vi "SLM CONTROL v2.vi"() -> ()   [LabVIEW 2014]
panel:
  out "Exit VI 2":bool
  in  "current metric":enum16{"brightness", "sharpness", "both"}(ring)
  in  "holo on 2":bool=TRUE
  in  "holo on 1":bool=TRUE
  in  "discard 1":bool
  in  "correct mode x 1":bool
  in  "mode x 1":i32=5 caption="x"
  in  "align tilt 1":bool
  in  "keep 1":bool
  in  "align tip 1":bool
  in  "discard 2":bool
  in  "correct mode x 2":bool
  in  "mode x 2":i32=5 caption="x"
  in  "align tilt 2":bool
  in  "keep 2":bool
  in  "fitted peak":dbl caption="x"
  in  "loop index":i32 caption="x"
  out "Metric Plots":cluster{dbl[], dbl[]}[](graph)
  in  "S Max":dbl=0.2 caption="x"
  in  "M":dbl[](array[numeric])=[0.0, 0.0]
  in  "BG Offset":dbl=0.2 caption="x"
  in  "Rmask":dbl=0.2 caption="x"
  in  "I":dbl[](array[numeric])=[0.0, 0.0, 0.0, 0.0, 0.0]
  in  "S":dbl[](array[numeric])=[0.0, 0.0, 0.0, 0.0, 0.0]
  in  "resolution":dbl=0.2 caption="x"
  out "current mode number":i32=5 caption="x"
  out "current holo number":i32=2 caption="x"
  in  "alignment offset":dbl[](array[numeric])=[0.0, 0.0]
  in  "step size align":dbl=0.2 caption="step size"
  in  "number of steps align":i32=3 caption="# steps"
  in  "align tip 2":bool
  in  "load BMP":bool
  in  "save hologram":bool
  in  "top hat radius":dbl=0.66
  out "mode matrix name":string="Unit Matrix.csv"
  in  "set mode matrix name":bool
  in  "holo size":i32=300
  in  "wrap value":i32=20
  in  "SLM number":i32=197
  in  "apply flatness":bool
  out "hologram":u8[][](graph)
  in  "vortex dir 2":bool
  in  "vortex dir 1":bool
  in  "top hat 2":bool
  in  "vortex 2":bool
  in  "top hat 1":bool
  in  "vortex 1":bool
  in  "holo y pos 2":dbl caption="y"
  in  "holo x pos 2":dbl=200.0 caption="x"
  in  "holo y pos 1":dbl caption="y"
  in  "holo x pos 1":dbl=-200.0 caption="x"
  in  "background gradient y":dbl=-40.0 caption="y"
  in  "background gradient x":dbl=-40.0 caption="x"
  in  "merlin coefficients 2":dbl[][](array[numeric])=[[0.0, 0.0], [0.0, 0.0], [0.0, 0.0]]
  in  "routine coefficients 2":dbl[][](array[numeric])=[[0.0, 0.0], [0.0, 0.0], [0.0, 0.0]]
  in  "manual coefficients 2":dbl[][](array[numeric])=[[2.0, 0.0], [3.0, 0.0], [4.0, 1.0]]
  in  "grating coefficients 2":dbl[][](array[numeric])=[[2.0, 0.0], [3.0, 0.0]]
  in  "merlin coefficients 1":dbl[][](array[numeric])=[[0.0, 0.0], [0.0, 0.0], [0.0, 0.0]]
  in  "routine coefficients 1":dbl[][](array[numeric])=[[0.0, 0.0], [0.0, 0.0], [0.0, 0.0]]
  in  "manual coefficients 1":dbl[][](array[numeric])=[[2.0, 0.0], [3.0, 0.0], [4.0, 1.0]]
  in  "grating coefficients 1":dbl[][](array[numeric])=[[2.0, 0.0], [3.0, 0.0]]
  in  "modes in memory":i32=20 caption="# modes"
  in  "wavelength (nm)":i32=197
  in  "max wavelength (nm)":i32=800
  in  "min wavelength (nm)":i32=700
  out "root path":path
  out "Sub VI Ready?":bool
  in  "Exit VI":bool
  # "Holo 1"
  # "Holo 2"
  # "Background"
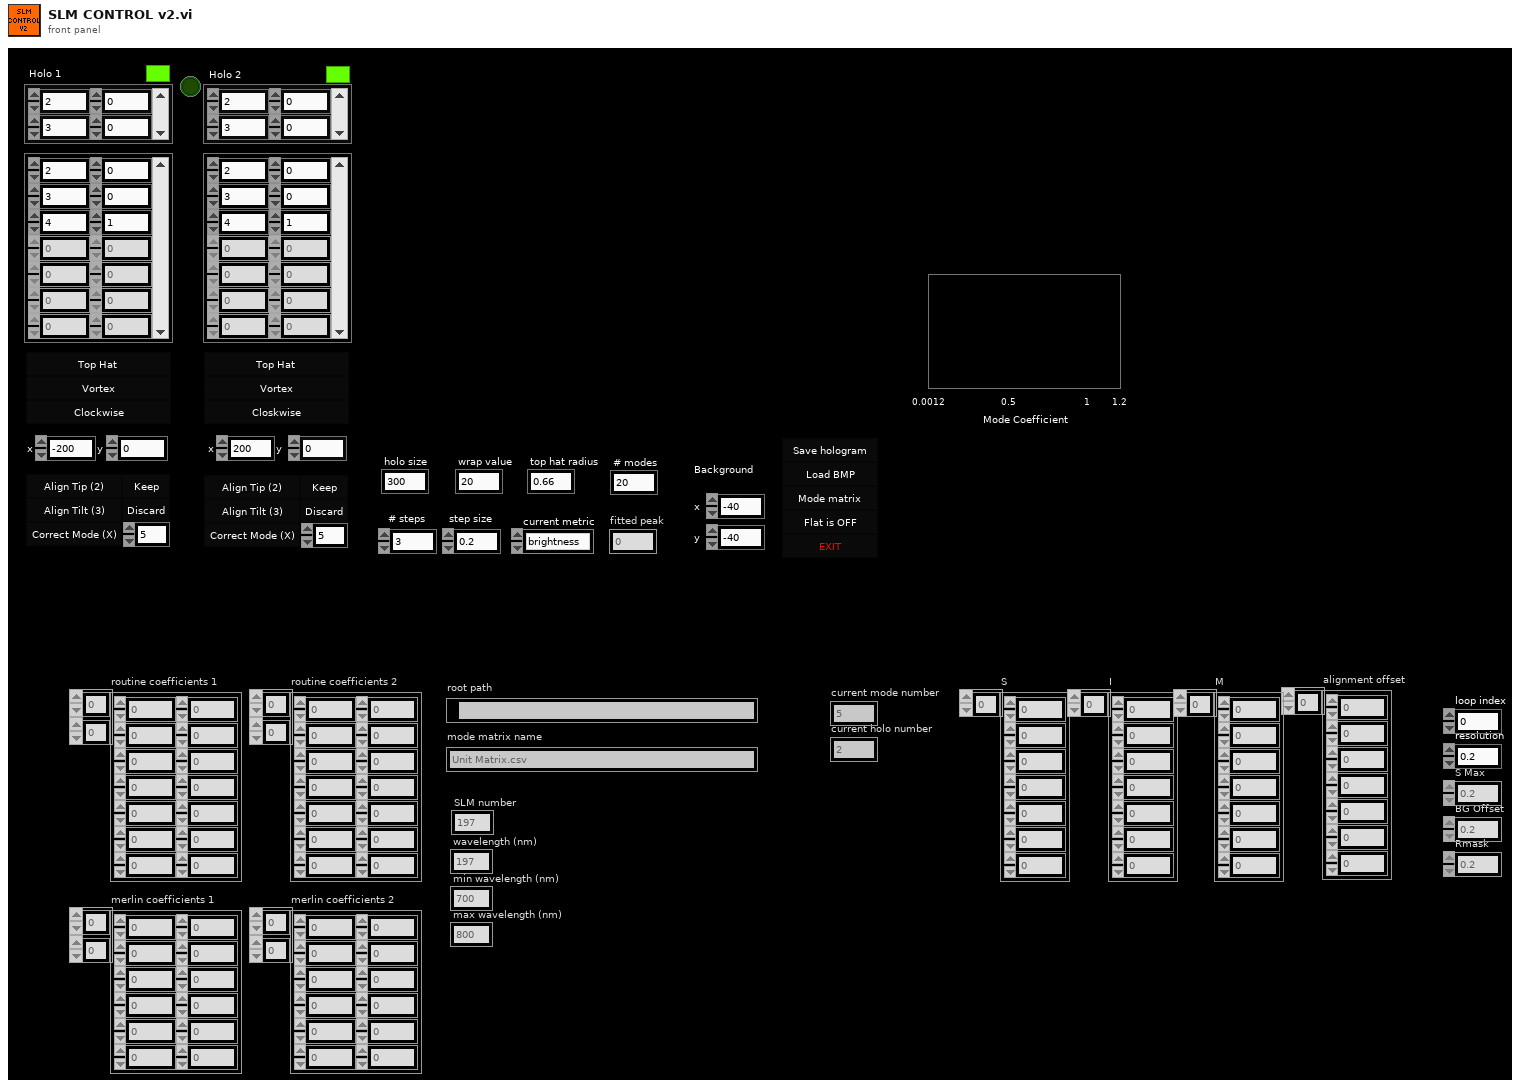
[diagram p1: front panel]
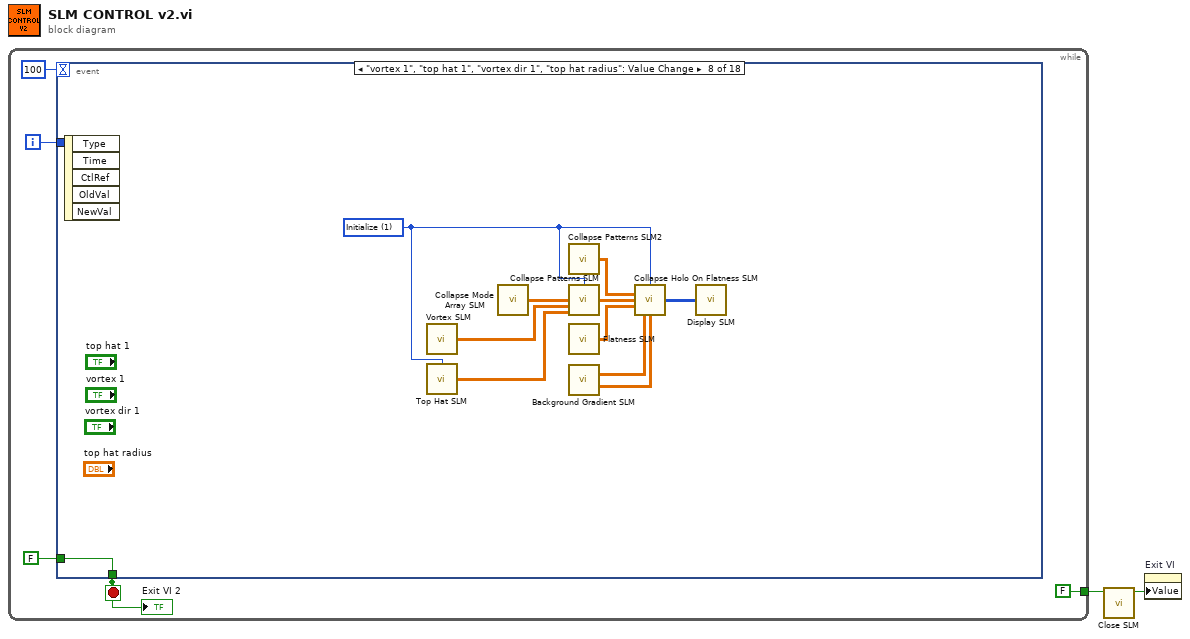
[diagram p0: block diagram]
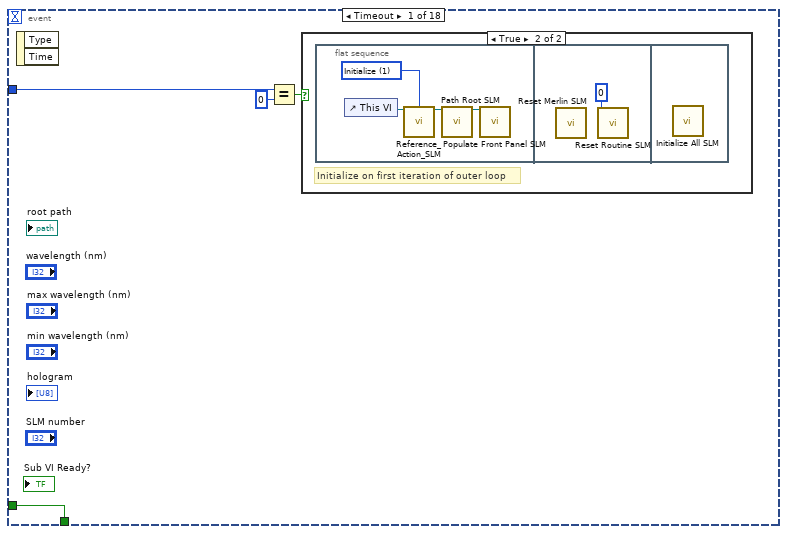
[diagram p2: hidden frame]
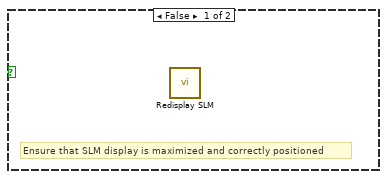
[diagram p3: hidden frame]
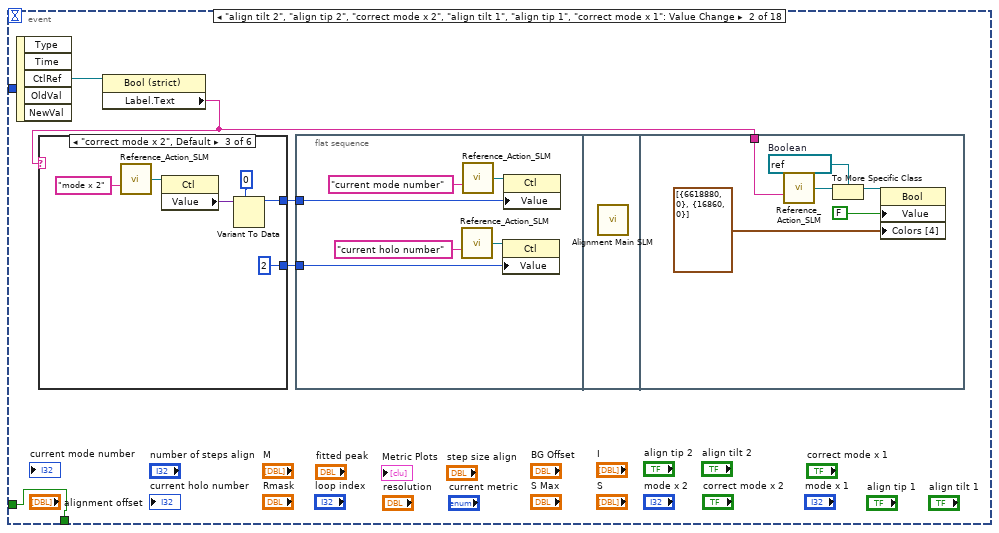
[diagram p4: hidden frame]
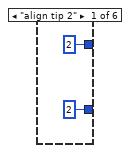
[diagram p5: hidden frame]
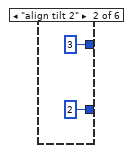
[diagram p6: hidden frame]
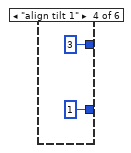
[diagram p7: hidden frame]
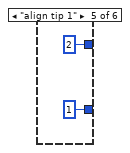
[diagram p8: hidden frame]
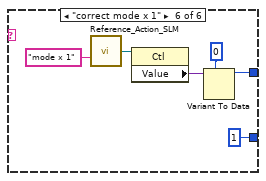
[diagram p9: hidden frame]
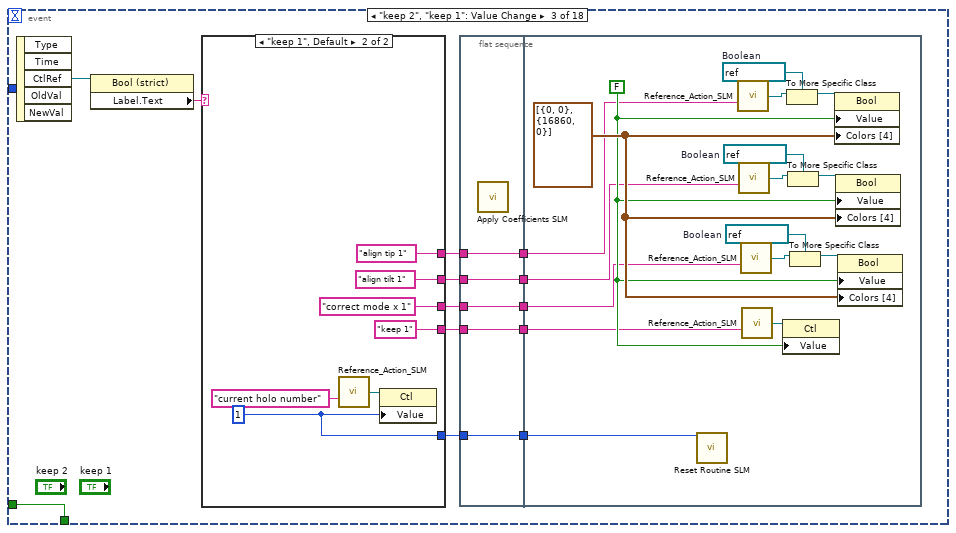
[diagram p10: hidden frame]
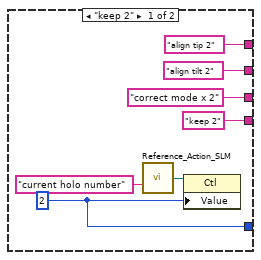
[diagram p11: hidden frame]
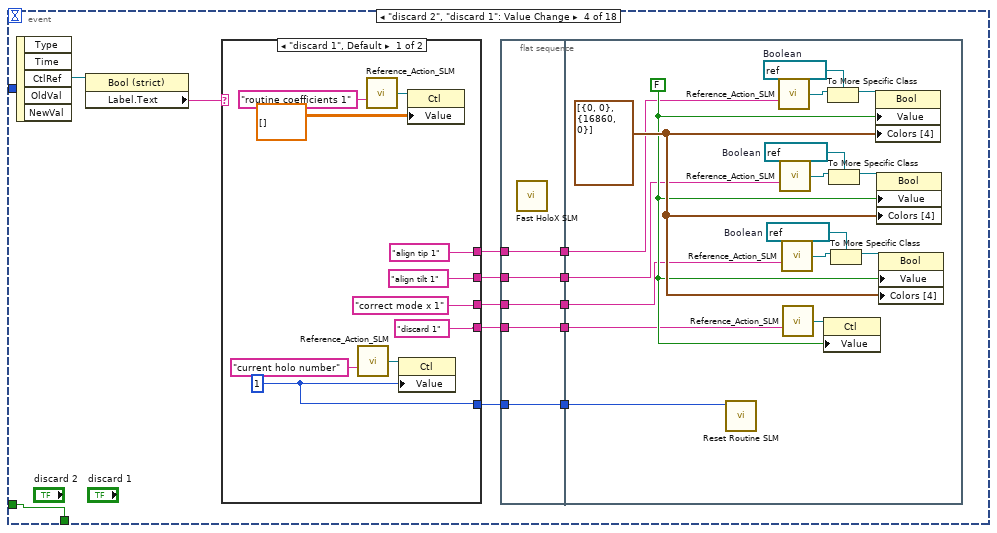
[diagram p12: hidden frame]
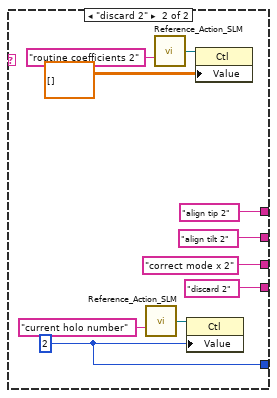
[diagram p13: hidden frame]
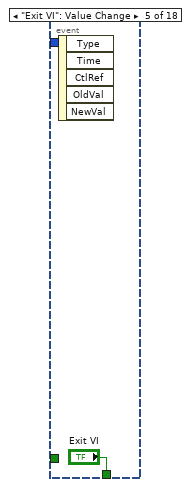
[diagram p14: hidden frame]
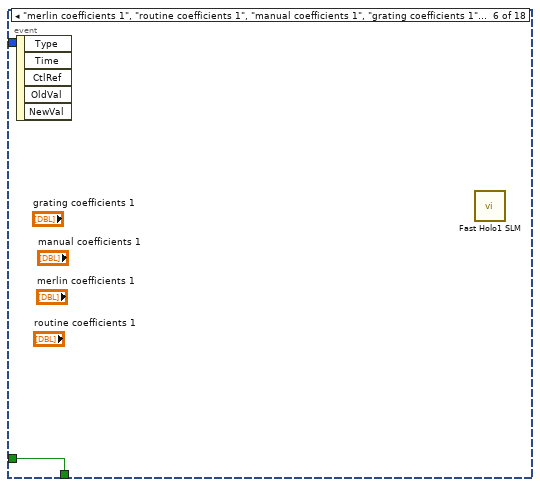
[diagram p15: hidden frame]
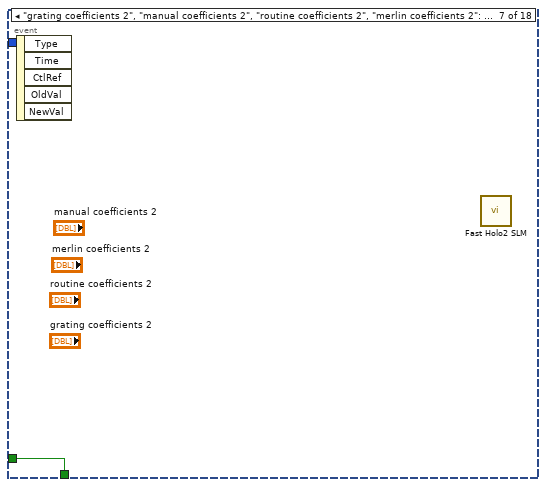
[diagram p16: hidden frame]
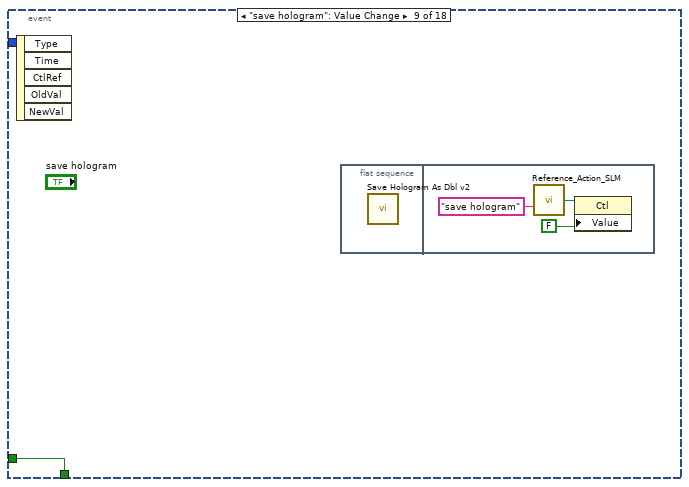
[diagram p17: hidden frame]
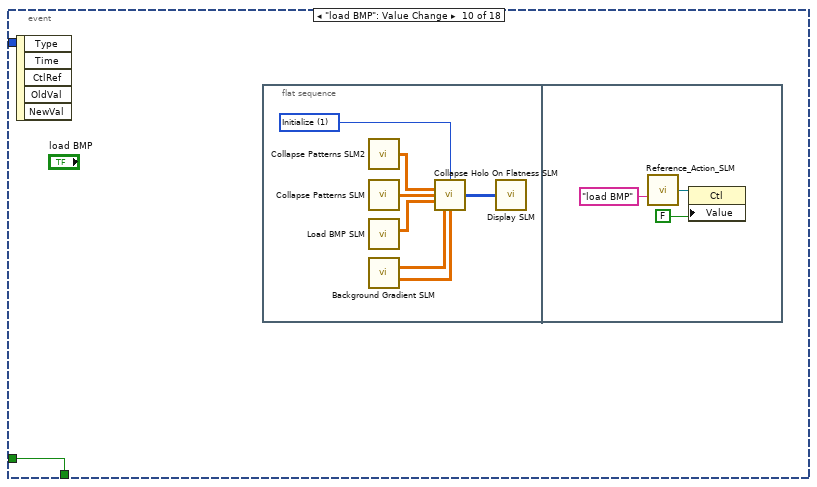
[diagram p18: hidden frame]
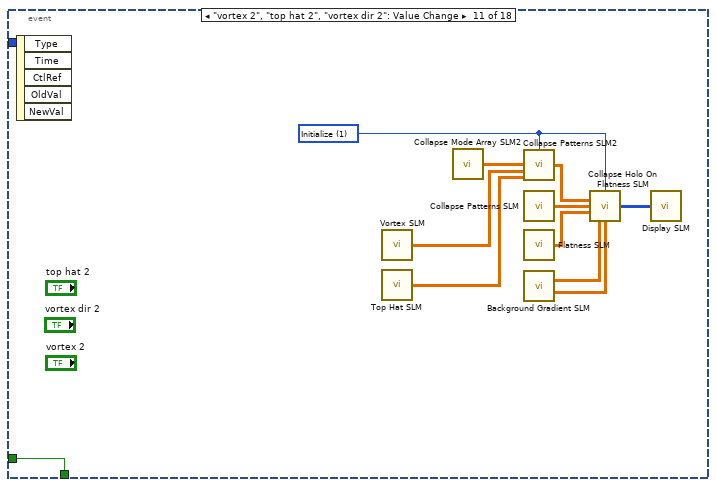
[diagram p19: hidden frame]
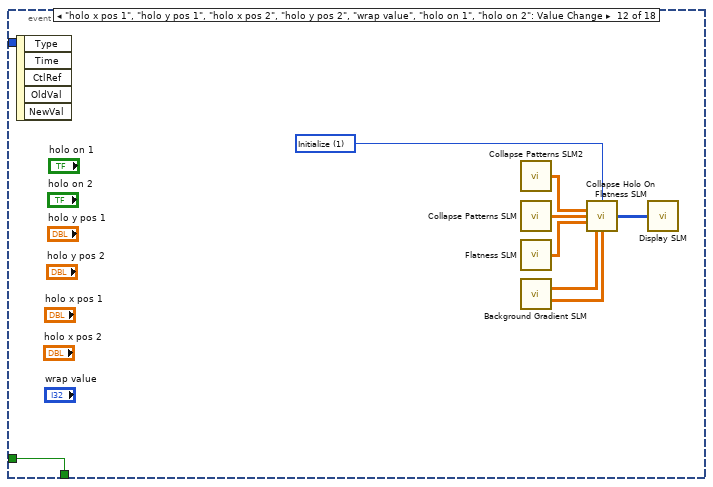
[diagram p20: hidden frame]
diagram:
  n1 = while {
    tunnel: [FALSE] -> w2
    i -> [w4]
    stop <- w7 stop-if-true
    n2 = event shown="[7] \"vortex 1\", \"top hat 1\", \"vortex dir 1\", \"top hat radius\": Value Change" {
      selector: _ -> [_ _ _ _ _ _ _ _ _ _ _ _ _ _ _ _ _ _]
      dyn-events: _ -> [_ _ _ _ _ _ _ _ _ _ _ _ _ _ _ _ _ _]
      timeout: 100 -> [_ _ _ _ _ _ _ _ _ _ _ _ _ _ _ _ _ _]
      tunnel: [w11 w17 w54 w103 "Exit VI" w159 w160 w161 w172 w176 w187 w198 w206 w214 w222 w235 w239 w244] -> w7
      tunnel: FALSE -> [w11 w17 w54 w103 _ w159 w160 w161 w172 w176 w187 w198 w206 w214 w222 w235 w239 w244]
      tunnel: w4 -> [w8 _ _ _ _ _ _ _ _ _ _ _ _ _ _ _ _ _]
      event Timeout {
        n3 = event-data() -> ()  [unwired: 3 out]
        n4 = Equal?(x=w8, y=0) -> (x = y?=w9:bool)
        n5 = case shown="True" w9 {
          frame False {
            # "Ensure that SLM display is maximized and correctly positioned"
            n6 = call "Redisplay SLM.vi"() -> ()  [unwired: 12 in]
          }
          frame True {
            # "Initialize on first iteration of outer loop"
            n7 = flat-sequence {
              frame #0 {
                w14 = u16 1 items=["Read", "Initialize"] ("Action")
                n8 = control-ref of="This VI"() -> (w13:refnum<vi>)
                n9 = call "Reference_Action_SLM.vi"("VI Ref IN"=w13, "Action"=w14) -> ("VI Reference"=w15:refnum<vi>)  [unwired: 11 in, 2 out]
                n10 = call "Path Root SLM.vi"("VI Ref IN"=w15) -> ("VI Ref OUT"=w12:refnum<vi>)  [unwired: 14 in]
                n11 = call "Populate Front Panel SLM.vi"("This VI"=w12) -> ()  [unwired: 11 in]
              }
              frame #1 {
                n12 = call "Reset Merlin SLM.vi"() -> ()  [unwired: 12 in]
                n13 = call "Reset Routine SLM.vi"("Numeric"=0) -> ()  [unwired: 11 in]
              }
              frame #2 {
                n14 = call "Initialize All SLM.vi"() -> ()  [unwired: 16 in]
              }
            }
          }
        }
      }
      event "align tilt 2", "align tip 2", "correct mode x 2", "align tilt 1", "align tip 1", "correct mode x 1": Value Change {
        n15 = event-data() -> ("CtlRef"=w21:refnum<vi>)  [unwired: 5 out]
        n16 = property class="Bool (strict)"(reference=w21) -> ("Label.Text"=w18:string)  [unwired: 1 in, 2 out]
        n17 = case shown="\"correct mode x 2\", Default" w18 {
          tunnel: [2 2 2 1 1 1] -> w20
          tunnel: [2 3 w27 3 2 w37] -> w19
          frame "align tip 2" {
          }
          frame "align tilt 2" {
          }
          frame "correct mode x 2", Default {
            n18 = call "Reference_Action_SLM.vi"("Control Name"="mode x 2") -> ("Ref OUT"=w29:refnum<vi>)  [unwired: 12 in, 2 out]
            n19 = property class="Ctl"(reference=w29) -> ("Value"=w30:variant)  [unwired: 1 in, 2 out]
            n20 = Variant To Data(type=0, Variant=w30) -> (data=w27:i32)  [unwired: 1 in, 1 out]
          }
          frame "align tilt 1" {
          }
          frame "align tip 1" {
          }
          frame "correct mode x 1" {
            n21 = call "Reference_Action_SLM.vi"("Control Name"="mode x 1") -> ("Ref OUT"=w39:refnum<vi>)  [unwired: 12 in, 2 out]
            n22 = property class="Ctl"(reference=w39) -> ("Value"=w40:variant)  [unwired: 1 in, 2 out]
            n23 = Variant To Data(type=0, Variant=w40) -> (data=w37:i32)  [unwired: 1 in, 1 out]
          }
        }
        n24 = flat-sequence {
          tunnel: w20 -> [w43]
          tunnel: w19 -> [w42]
          tunnel: w18 -> [w48]
          frame #0 {
            n25 = call "Reference_Action_SLM.vi"("Control Name"="current holo number") -> ("Ref OUT"=w44:refnum<vi>)  [unwired: 12 in, 2 out]
            n26 = call "Reference_Action_SLM.vi"("Control Name"="current mode number") -> ("Ref OUT"=w46:refnum<vi>)  [unwired: 12 in, 2 out]
            n27 = property class="Ctl"(reference=w44, "Value"=w43) -> ()  [unwired: 1 in, 2 out]
            n28 = property class="Ctl"(reference=w46, "Value"=w42) -> ()  [unwired: 1 in, 2 out]
          }
          frame #1 {
            n29 = call "Alignment Main SLM.vi"() -> ()  [unwired: 12 in]
          }
          frame #2 {
            w51 = refnum<vi> refnum  # Boolean
            n30 = call "Reference_Action_SLM.vi"("Control Name"=w48) -> ("Ref OUT"=w53:refnum<vi>)  [unwired: 12 in, 2 out]
            n31 = To More Specific Class(target class=w51, reference=w53) -> (specific class reference=w52:refnum<vi>)  [unwired: 1 in, 1 out]
            n32 = property class="Bool"(reference=w52, "Value"=FALSE, "Colors [4]"=cluster{u32, u32}[] [{6618880, 0}, {16860, 0}]) -> ()  [unwired: 1 in, 2 out]
          }
        }
      }
      event "keep 2", "keep 1": Value Change {
        n33 = event-data() -> ("CtlRef"=w66:refnum<vi>)  [unwired: 5 out]
        n34 = property class="Bool (strict)"(reference=w66) -> ("Label.Text"=w65:string)  [unwired: 1 in, 2 out]
        n35 = case shown="\"keep 1\", Default" w65 {
          tunnel: ["keep 2" ("Control Name") "keep 1" ("Control Name")] -> w63
          tunnel: ["correct mode x 2" ("Control Name") "correct mode x 1" ("Control Name")] -> w61
          tunnel: ["align tilt 2" ("Control Name") "align tilt 1" ("Control Name")] -> w59
          tunnel: ["align tip 2" ("Control Name") "align tip 1" ("Control Name")] -> w57
          tunnel: [w67 w74] -> w55
          frame "keep 2" {
            w67 = 2
            n36 = call "Reference_Action_SLM.vi"("Control Name"="current holo number") -> ("Ref OUT"=w69:refnum<vi>)  [unwired: 12 in, 2 out]
            n37 = property class="Ctl"(reference=w69, "Value"=w67) -> ()  [unwired: 1 in, 2 out]
          }
          frame "keep 1", Default {
            w74 = 1
            n38 = call "Reference_Action_SLM.vi"("Control Name"="current holo number") -> ("Ref OUT"=w76:refnum<vi>)  [unwired: 12 in, 2 out]
            n39 = property class="Ctl"(reference=w76, "Value"=w74) -> ()  [unwired: 1 in, 2 out]
          }
        }
        n40 = flat-sequence {
          tunnel: [w85] -> w64
          tunnel: w63 -> [w85]
          tunnel: [w84] -> w62
          tunnel: w61 -> [w84]
          tunnel: [w83] -> w60
          tunnel: w59 -> [w83]
          tunnel: [w82] -> w58
          tunnel: w57 -> [w82]
          tunnel: [w81] -> w56
          tunnel: w55 -> [w81]
          tunnel: w64 -> [w90]
          tunnel: w62 -> [w89]
          tunnel: w60 -> [w88]
          tunnel: w58 -> [w87]
          tunnel: w56 -> [w86]
          frame #0 {
            n41 = call "Apply Coefficients SLM.vi"() -> ()  [unwired: 12 in]
          }
          frame #1 {
            w93 = refnum<vi> refnum  # Boolean
            w92 = cluster{u32, u32}[] [{0, 0}, {16860, 0}] ("Colors [4]")
            w96 = refnum<vi> refnum  # Boolean
            w91 = FALSE
            w99 = refnum<vi> refnum  # Boolean
            n42 = call "Reset Routine SLM.vi"("Numeric"=w86) -> ()  [unwired: 11 in]
            n43 = call "Reference_Action_SLM.vi"("Control Name"=w87) -> ("Ref OUT"=w101:refnum<vi>)  [unwired: 12 in, 2 out]
            n44 = call "Reference_Action_SLM.vi"("Control Name"=w88) -> ("Ref OUT"=w98:refnum<vi>)  [unwired: 12 in, 2 out]
            n45 = call "Reference_Action_SLM.vi"("Control Name"=w89) -> ("Ref OUT"=w95:refnum<vi>)  [unwired: 12 in, 2 out]
            n46 = call "Reference_Action_SLM.vi"("Control Name"=w90) -> ("Ref OUT"=w102:refnum<vi>)  [unwired: 12 in, 2 out]
            n47 = property class="Ctl"(reference=w102, "Value"=w91) -> ()  [unwired: 1 in, 2 out]
            n48 = To More Specific Class(target class=w99, reference=w101) -> (specific class reference=w100:refnum<vi>)  [unwired: 1 in, 1 out]
            n49 = To More Specific Class(target class=w96, reference=w98) -> (specific class reference=w97:refnum<vi>)  [unwired: 1 in, 1 out]
            n50 = To More Specific Class(target class=w93, reference=w95) -> (specific class reference=w94:refnum<vi>)  [unwired: 1 in, 1 out]
            n51 = property class="Bool"(reference=w100, "Value"=w91, "Colors [4]"=w92) -> ()  [unwired: 1 in, 2 out]
            n52 = property class="Bool"(reference=w97, "Value"=w91, "Colors [4]"=w92) -> ()  [unwired: 1 in, 2 out]
            n53 = property class="Bool"(reference=w94, "Value"=w91, "Colors [4]"=w92) -> ()  [unwired: 1 in, 2 out]
          }
        }
      }
      event "discard 2", "discard 1": Value Change {
        n54 = event-data() -> ("CtlRef"=w115:refnum<vi>)  [unwired: 5 out]
        n55 = property class="Bool (strict)"(reference=w115) -> ("Label.Text"=w114:string)  [unwired: 1 in, 2 out]
        n56 = case shown="\"discard 1\", Default" w114 {
          tunnel: ["discard 1" ("Control Name") "discard 2" ("Control Name")] -> w106
          tunnel: ["correct mode x 1" ("Control Name") "correct mode x 2" ("Control Name")] -> w107
          tunnel: ["align tilt 1" ("Control Name") "align tilt 2" ("Control Name")] -> w108
          tunnel: ["align tip 1" ("Control Name") "align tip 2" ("Control Name")] -> w109
          tunnel: [w138 w148] -> w104
          frame "discard 1", Default {
            w138 = 1
            n57 = call "Reference_Action_SLM.vi"("Control Name"="current holo number") -> ("Ref OUT"=w144:refnum<vi>)  [unwired: 12 in, 2 out]
            n58 = call "Reference_Action_SLM.vi"("Control Name"="routine coefficients 1") -> ("Ref OUT"=w145:refnum<vi>)  [unwired: 12 in, 2 out]
            n59 = property class="Ctl"(reference=w144, "Value"=w138) -> ()  [unwired: 1 in, 2 out]
            n60 = property class="Ctl"(reference=w145, "Value"=dbl[][] [] ("routine coefficients 2")) -> ()  [unwired: 1 in, 2 out]
          }
          frame "discard 2" {
            w148 = 2
            n61 = call "Reference_Action_SLM.vi"("Control Name"="current holo number") -> ("Ref OUT"=w150:refnum<vi>)  [unwired: 12 in, 2 out]
            n62 = call "Reference_Action_SLM.vi"("Control Name"="routine coefficients 2") -> ("Ref OUT"=w151:refnum<vi>)  [unwired: 12 in, 2 out]
            n63 = property class="Ctl"(reference=w150, "Value"=w148) -> ()  [unwired: 1 in, 2 out]
            n64 = property class="Ctl"(reference=w151, "Value"=dbl[][] [] ("routine coefficients 2")) -> ()  [unwired: 1 in, 2 out]
          }
        }
        n65 = flat-sequence {
          tunnel: [w120] -> w113
          tunnel: w106 -> [w120]
          tunnel: [w119] -> w112
          tunnel: w107 -> [w119]
          tunnel: [w118] -> w111
          tunnel: w108 -> [w118]
          tunnel: [w117] -> w110
          tunnel: w109 -> [w117]
          tunnel: [w116] -> w105
          tunnel: w104 -> [w116]
          tunnel: w113 -> [w125]
          tunnel: w112 -> [w124]
          tunnel: w111 -> [w123]
          tunnel: w110 -> [w122]
          tunnel: w105 -> [w121]
          frame #0 {
            n66 = call "Fast HoloX SLM.vi"() -> ()  [unwired: 12 in]
          }
          frame #1 {
            w128 = refnum<vi> refnum  # Boolean
            w127 = cluster{u32, u32}[] [{0, 0}, {16860, 0}] ("Colors [4]")
            w131 = refnum<vi> refnum  # Boolean
            w126 = FALSE
            w134 = refnum<vi> refnum  # Boolean
            n67 = call "Reset Routine SLM.vi"("Numeric"=w121) -> ()  [unwired: 11 in]
            n68 = call "Reference_Action_SLM.vi"("Control Name"=w122) -> ("Ref OUT"=w136:refnum<vi>)  [unwired: 12 in, 2 out]
            n69 = call "Reference_Action_SLM.vi"("Control Name"=w123) -> ("Ref OUT"=w133:refnum<vi>)  [unwired: 12 in, 2 out]
            n70 = call "Reference_Action_SLM.vi"("Control Name"=w124) -> ("Ref OUT"=w130:refnum<vi>)  [unwired: 12 in, 2 out]
            n71 = call "Reference_Action_SLM.vi"("Control Name"=w125) -> ("Ref OUT"=w137:refnum<vi>)  [unwired: 12 in, 2 out]
            n72 = property class="Ctl"(reference=w137, "Value"=w126) -> ()  [unwired: 1 in, 2 out]
            n73 = To More Specific Class(target class=w134, reference=w136) -> (specific class reference=w135:refnum<vi>)  [unwired: 1 in, 1 out]
            n74 = To More Specific Class(target class=w131, reference=w133) -> (specific class reference=w132:refnum<vi>)  [unwired: 1 in, 1 out]
            n75 = To More Specific Class(target class=w128, reference=w130) -> (specific class reference=w129:refnum<vi>)  [unwired: 1 in, 1 out]
            n76 = property class="Bool"(reference=w135, "Value"=w126, "Colors [4]"=w127) -> ()  [unwired: 1 in, 2 out]
            n77 = property class="Bool"(reference=w132, "Value"=w126, "Colors [4]"=w127) -> ()  [unwired: 1 in, 2 out]
            n78 = property class="Bool"(reference=w129, "Value"=w126, "Colors [4]"=w127) -> ()  [unwired: 1 in, 2 out]
          }
        }
      }
      event "Exit VI": Value Change {
        n79 = event-data() -> ()  [unwired: 6 out]
      }
      event "merlin coefficients 1", "routine coefficients 1", "manual coefficients 1", "grating coefficients 1": Value Change {
        n80 = event-data() -> ()  [unwired: 6 out]
        n81 = call "Fast Holo1 SLM.vi"() -> ()  [unwired: 12 in]
      }
      event "grating coefficients 2", "manual coefficients 2", "routine coefficients 2", "merlin coefficients 2": Value Change {
        n82 = event-data() -> ()  [unwired: 6 out]
        n83 = call "Fast Holo2 SLM.vi"() -> ()  [unwired: 12 in]
      }
      event "vortex 1", "top hat 1", "vortex dir 1", "top hat radius": Value Change {
        w162 = u16 1 items=["Read", "Initialize"] ("Action")
        n84 = event-data() -> ()  [unwired: 6 out]
        n85 = call "Vortex SLM.vi"() -> ("Vortex"=w169:dbl[][])  [unwired: 15 in]
        n86 = call "Top Hat SLM.vi"("Action"=w162) -> ("Top hat"=w168:dbl[][])  [unwired: 14 in]
        n87 = call "Collapse Mode Array SLM.vi"() -> ("collapsed mode array"=w171:dbl[][])  [unwired: 15 in]
        n88 = call "Collapse Patterns SLM2.vi"() -> ("collapsed patterns"=w165:dbl[][])  [unwired: 15 in]
        n89 = call "Collapse Patterns SLM.vi"("Action"=w162, "collapsed mode array"=w171, "Vortex"=w169, "Top hat"=w168) -> ("collapsed patterns"=w170:dbl[][])  [unwired: 11 in]
        n90 = call "Flatness SLM.vi"() -> ("flatness"=w167:dbl[][])  [unwired: 15 in]
        n91 = call "Background Gradient SLM.vi"() -> ("gradient"=w164:dbl[][], "holo mask"=w163:dbl[][])  [unwired: 14 in]
        n92 = call "Collapse Holo On Flatness SLM.vi"("Action"=w162, "collapsed patterns 2"=w165, "collapsed patterns"=w170, "flatness"=w167, "gradient"=w164, "holo mask"=w163) -> ("displayed matrix"=w166:u8[][])  [unwired: 9 in]
        n93 = call "Display SLM.vi"("displayed matrix"=w166) -> ()  [unwired: 14 in, 1 out]
      }
      event "save hologram": Value Change {
        n94 = event-data() -> ()  [unwired: 6 out]
        n95 = flat-sequence {
          frame #0 {
            n96 = call "Save Hologram As Dbl v2.vi"() -> ()  [unwired: 12 in]
          }
          frame #1 {
            n97 = call "Reference_Action_SLM.vi"("Control Name"="save hologram") -> ("Ref OUT"=w174:refnum<vi>)  [unwired: 12 in, 2 out]
            n98 = property class="Ctl"(reference=w174, "Value"=FALSE ("Load Matrix")) -> ()  [unwired: 1 in, 2 out]
          }
        }
      }
      event "load BMP": Value Change {
        n99 = event-data() -> ()  [unwired: 6 out]
        n100 = flat-sequence {
          frame #0 {
            w178 = u16 1 items=["Read", "Initialize"] ("Action")
            n101 = call "Collapse Patterns SLM2.vi"() -> ("collapsed patterns"=w181:dbl[][])  [unwired: 15 in]
            n102 = call "Collapse Patterns SLM.vi"() -> ("collapsed patterns"=w183:dbl[][])  [unwired: 15 in]
            n103 = call "Load BMP SLM.vi"() -> ("double precision float"=w177:dbl[][])  [unwired: 11 in]
            n104 = call "Background Gradient SLM.vi"() -> ("gradient"=w180:dbl[][], "holo mask"=w179:dbl[][])  [unwired: 14 in]
            n105 = call "Collapse Holo On Flatness SLM.vi"("Action"=w178, "collapsed patterns 2"=w181, "collapsed patterns"=w183, "flatness"=w177, "gradient"=w180, "holo mask"=w179) -> ("displayed matrix"=w182:u8[][])  [unwired: 9 in]
            n106 = call "Display SLM.vi"("displayed matrix"=w182) -> ()  [unwired: 14 in, 1 out]
          }
          frame #1 {
            n107 = call "Reference_Action_SLM.vi"("Control Name"="load BMP") -> ("Ref OUT"=w185:refnum<vi>)  [unwired: 12 in, 2 out]
            n108 = property class="Ctl"(reference=w185, "Value"=FALSE ("Load Matrix")) -> ()  [unwired: 1 in, 2 out]
          }
        }
      }
      event "vortex 2", "top hat 2", "vortex dir 2": Value Change {
        w193 = u16 1 items=["Read", "Initialize"] ("Action")
        n109 = event-data() -> ()  [unwired: 6 out]
        n110 = call "Vortex SLM.vi"() -> ("Vortex"=w191:dbl[][])  [unwired: 15 in]
        n111 = call "Top Hat SLM.vi"() -> ("Top hat"=w190:dbl[][])  [unwired: 15 in]
        n112 = call "Collapse Mode Array SLM2.vi"() -> ("collapsed mode array"=w192:dbl[][])  [unwired: 15 in]
        n113 = call "Collapse Patterns SLM2.vi"("Action"=w193, "collapsed mode array"=w192, "Vortex"=w191, "Top hat"=w190) -> ("collapsed patterns"=w194:dbl[][])  [unwired: 11 in]
        n114 = call "Collapse Patterns SLM.vi"() -> ("collapsed patterns"=w197:dbl[][])  [unwired: 15 in]
        n115 = call "Flatness SLM.vi"() -> ("flatness"=w196:dbl[][])  [unwired: 15 in]
        n116 = call "Background Gradient SLM.vi"() -> ("gradient"=w189:dbl[][], "holo mask"=w188:dbl[][])  [unwired: 14 in]
        n117 = call "Collapse Holo On Flatness SLM.vi"("Action"=w193, "collapsed patterns 2"=w194, "collapsed patterns"=w197, "flatness"=w196, "gradient"=w189, "holo mask"=w188) -> ("displayed matrix"=w195:u8[][])  [unwired: 9 in]
        n118 = call "Display SLM.vi"("displayed matrix"=w195) -> ()  [unwired: 14 in, 1 out]
      }
      event "holo x pos 1", "holo y pos 1", "holo x pos 2", "holo y pos 2", "wrap value", "holo on 1", "holo on 2": Value Change {
        w205 = u16 1 items=["Read", "Initialize"] ("Action")
        n119 = event-data() -> ()  [unwired: 6 out]
        n120 = call "Collapse Patterns SLM2.vi"() -> ("collapsed patterns"=w201:dbl[][])  [unwired: 15 in]
        n121 = call "Collapse Patterns SLM.vi"() -> ("collapsed patterns"=w202:dbl[][])  [unwired: 15 in]
        n122 = call "Flatness SLM.vi"() -> ("flatness"=w203:dbl[][])  [unwired: 15 in]
        n123 = call "Background Gradient SLM.vi"() -> ("gradient"=w200:dbl[][], "holo mask"=w199:dbl[][])  [unwired: 14 in]
        n124 = call "Collapse Holo On Flatness SLM.vi"("Action"=w205, "collapsed patterns 2"=w201, "collapsed patterns"=w202, "flatness"=w203, "gradient"=w200, "holo mask"=w199) -> ("displayed matrix"=w204:u8[][])  [unwired: 9 in]
        n125 = call "Display SLM.vi"("displayed matrix"=w204) -> ()  [unwired: 14 in, 1 out]
      }
      event "background gradient x", "background gradient y": Value Change {
        w208 = u16 1 items=["Read", "Initialize"] ("Action")
        n126 = event-data() -> ()  [unwired: 6 out]
        n127 = call "Collapse Patterns SLM2.vi"() -> ("collapsed patterns"=w210:dbl[][])  [unwired: 15 in]
        n128 = call "Collapse Patterns SLM.vi"() -> ("collapsed patterns"=w211:dbl[][])  [unwired: 15 in]
        n129 = call "Flatness SLM.vi"() -> ("flatness"=w212:dbl[][])  [unwired: 15 in]
        n130 = call "Background Gradient SLM.vi"("Action"=w208) -> ("gradient"=w209:dbl[][], "holo mask"=w207:dbl[][])  [unwired: 13 in]
        n131 = call "Collapse Holo On Flatness SLM.vi"("Action"=w208, "collapsed patterns 2"=w210, "collapsed patterns"=w211, "flatness"=w212, "gradient"=w209, "holo mask"=w207) -> ("displayed matrix"=w213:u8[][])  [unwired: 9 in]
        n132 = call "Display SLM.vi"("displayed matrix"=w213) -> ()  [unwired: 14 in, 1 out]
      }
      event "apply flatness": Value Change {
        w215 = u16 1 items=["Read", "Initialize"] ("Action")
        n133 = event-data() -> ()  [unwired: 6 out]
        n134 = call "Collapse Patterns SLM2.vi"() -> ("collapsed patterns"=w218:dbl[][])  [unwired: 15 in]
        n135 = call "Collapse Patterns SLM.vi"() -> ("collapsed patterns"=w219:dbl[][])  [unwired: 15 in]
        n136 = call "Flatness SLM.vi"("Action"=w215) -> ("flatness"=w220:dbl[][])  [unwired: 14 in]
        n137 = call "Background Gradient SLM.vi"() -> ("gradient"=w217:dbl[][], "holo mask"=w216:dbl[][])  [unwired: 14 in]
        n138 = call "Collapse Holo On Flatness SLM.vi"("Action"=w215, "collapsed patterns 2"=w218, "collapsed patterns"=w219, "flatness"=w220, "gradient"=w217, "holo mask"=w216) -> ("displayed matrix"=w221:u8[][])  [unwired: 9 in]
        n139 = call "Display SLM.vi"("displayed matrix"=w221) -> ()  [unwired: 14 in, 1 out]
      }
      event "holo size", "modes in memory": Value Change {
        w223 = u16 1 items=["Read", "Initialize"] ("Action")
        n140 = event-data() -> ()  [unwired: 6 out]
        n141 = call "Mode Array SLM.vi"("Action"=w223) -> ("mode array"=w230:dbl[][][])  [unwired: 14 in]
        n142 = call "Vortex SLM.vi"("Action"=w223) -> ("Vortex"=w228:dbl[][])  [unwired: 14 in]
        n143 = call "Top Hat SLM.vi"("Action"=w223) -> ("Top hat"=w227:dbl[][])  [unwired: 14 in]
        n144 = call "Collapse Mode Array SLM2.vi"("Action"=w223, "mode array"=w230) -> ("collapsed mode array"=w229:dbl[][])  [unwired: 13 in]
        n145 = call "Collapse Mode Array SLM.vi"("Action"=w223, "mode array"=w230) -> ("collapsed mode array"=w231:dbl[][])  [unwired: 13 in]
        n146 = call "Collapse Patterns SLM.vi"("Action"=w223, "collapsed mode array"=w231, "Vortex"=w228, "Top hat"=w227) -> ("collapsed patterns"=w232:dbl[][])  [unwired: 11 in]
        n147 = call "Flatness SLM.vi"() -> ("flatness"=w233:dbl[][])  [unwired: 15 in]
        n148 = call "Background Gradient SLM.vi"("Action"=w223) -> ("gradient"=w225:dbl[][], "holo mask"=w224:dbl[][])  [unwired: 13 in]
        n149 = call "Collapse Patterns SLM2.vi"("Action"=w223, "collapsed mode array"=w229, "Vortex"=w228, "Top hat"=w227) -> ("collapsed patterns"=w226:dbl[][])  [unwired: 11 in]
        n150 = call "Collapse Holo On Flatness SLM.vi"("Action"=w223, "collapsed patterns 2"=w226, "collapsed patterns"=w232, "flatness"=w233, "gradient"=w225, "holo mask"=w224) -> ("displayed matrix"=w234:u8[][])  [unwired: 9 in]
        n151 = call "Display SLM.vi"("displayed matrix"=w234) -> ()  [unwired: 14 in, 1 out]
      }
      event "set mode matrix name": Value Change {
        n152 = event-data() -> ()  [unwired: 6 out]
        n153 = flat-sequence {
          frame #0 {
            n154 = call "Mode Matrix Name SLM.vi"() -> ()  [unwired: 12 in]
          }
          frame #1 {
            n155 = call "Initialize All SLM.vi"() -> ()  [unwired: 16 in]
          }
          frame #2 {
            n156 = call "Reference_Action_SLM.vi"("Control Name"="set mode matrix name") -> ("Ref OUT"=w237:refnum<vi>)  [unwired: 12 in, 2 out]
            n157 = property class="Ctl"(reference=w237, "Value"=FALSE ("Load Matrix")) -> ()  [unwired: 1 in, 2 out]
          }
        }
      }
      event "Metric Plots": Mouse Down {
        n158 = event-data() -> ()  [unwired: 8 out]
        n159 = call "Reference_Action_SLM.vi"("Control Name"="Metric Plots") -> ("Ref OUT"=w240:refnum<vi>)  [unwired: 12 in, 2 out]
        n160 = property on="Property Node" class="Ctl"(reference=w240, "Left"=900 ("Position:Left"), "Top"=208 ("Position:Top")) -> ()  [unwired: 1 in, 2 out]
      }
      event "current metric": Value Change {
        n161 = event-data() -> ()  [unwired: 6 out]
        n162 = flat-sequence {
          frame #0 {
            n163 = call "Fit and Plot Metric v2.vi"() -> ("Peak"=w245:dbl)  [unwired: 11 in]
            n164 = call "Alignment Apply Offset SLM.vi"("current offset"=w245) -> ()  [unwired: 11 in]
          }
          frame #1 {
            n165 = call "Fast HoloX SLM.vi"() -> ()  [unwired: 12 in]
          }
        }
      }
    }
    "Exit VI 2" <- w7
  }
  n166 = call "Close SLM.vi"("Boolean"=w2) -> ("Boolean 2"=w1:bool)  [unwired: 10 in]
  n167 = property on="Exit VI" class="Bool (strict)"("Value"=w1) -> ()  [unwired: 2 in, 2 out]
